vi "获取paticle中心坐标.vi"(11 "Particle Measurements (Pixels) (Particle Analysis 1)":dbl[][](array[numeric])) -> (3 "数组":cluster{"Numeric":dbl, "Numeric":dbl}[](array[cluster]))   [LabVIEW 2014]
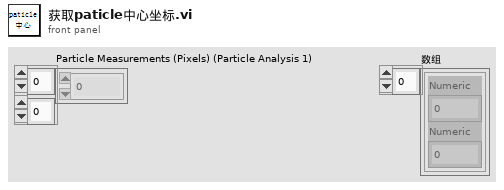
[diagram p1: front panel]
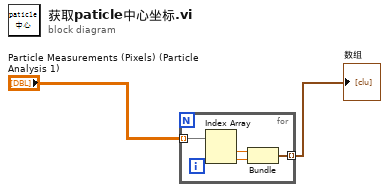
[diagram p0: block diagram]
diagram:
  n1 = for {
    tunnel: "Particle Measurements (Pixels) (Particle Analysis 1)" -> [w4] mode=indexing
    tunnel: [w3] -> w2 mode=indexing
    n2 = Index Array(array=w4) -> (element #1=w5:dbl, element #2=w6:dbl)  [unwired: 2 in]
    n3 = Bundle("Numeric"=w5, "Numeric"=w6) -> (w3:cluster{"Numeric":dbl, "Numeric":dbl})  [unwired: 1 in]
  }
  "数组" <- w2
